vi "WLAN - RxMeasure - DLL - VI.vi"() -> ()   [LabVIEW 2012]
panel:
  out "error out 4":errorcluster
  in  "Path Loss":dbl
  in  "RxPower":dbl
  in  "RF:Frequency (Hz)":dbl
  out "error out 2":errorcluster
  out "error out":errorcluster
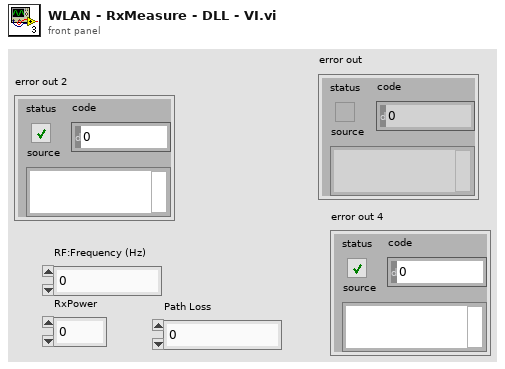
[diagram p1: front panel]
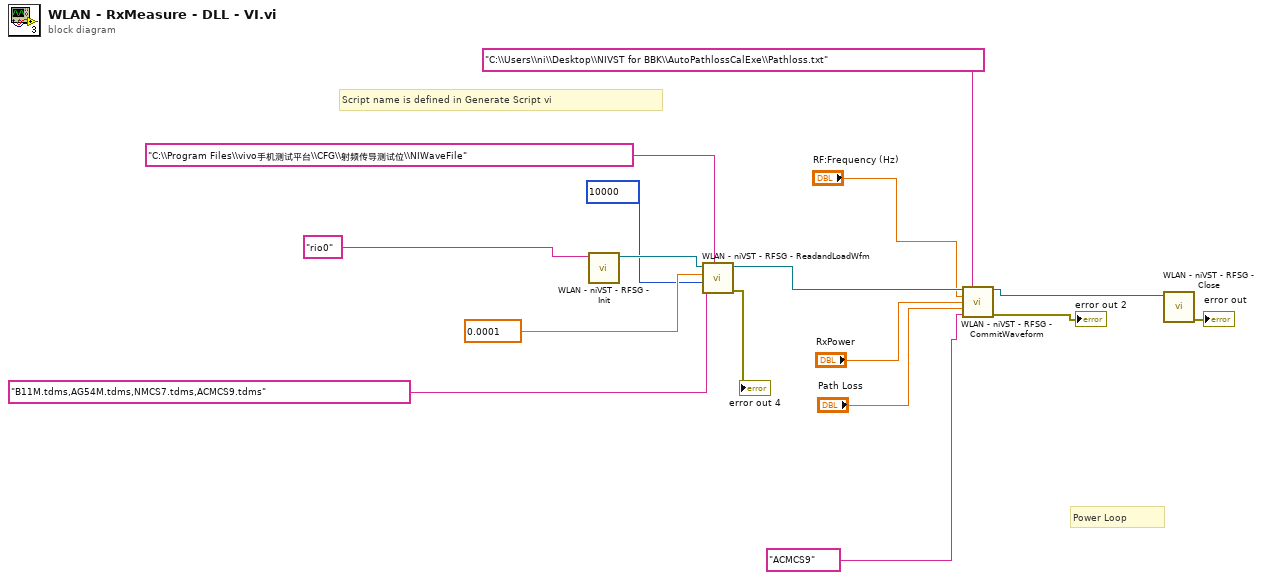
[diagram p0: block diagram]
diagram:
  # "Power Loop"
  # "Script name is defined in Generate Script vi"
  n1 = call "WLAN - niVST - RFSG - Init.vi"("RFSG Handle In"="rio0" ("RFSG Handle")) -> ("RFSG handle Out"=w12:refnum<k15>)  [unwired: 9 in, 1 out]
  n2 = call "WLAN - niVST - RFSG - ReadandLoadWfm.vi"("WfmFolderPath"="C:\\Program Files\\vivo手机测试平台\\CFG\\射频传导测试位\\NIWaveFile", "AllRxWfmName"="B11M.tdms,AG54M.tdms,NMCS7.tdms,ACMCS9.tdms", "numPackets"=10000 ("Number of Packets"), "Idle Time (With Ack)"=0.0001, "RFSG Handle In"=w12) -> ("error out"=→"error out 4":errorcluster, "RFSG Handle Out"=w9:refnum<k15>)  [unwired: 5 in]
  n3 = call "WLAN - niVST - RFSG - CommitWaveform.vi"("RFSG Handle In"=w9, "Internal pathloss file"="C:\\Users\\ni\\Desktop\\NIVST for BBK\\AutoPathlossCalExe\\Pathloss.txt", "RF:Frequency (Hz)"="RF:Frequency (Hz)", "RxPower"="RxPower", "External Path Loss"="Path Loss", "WfmName"="ACMCS9") -> ("RFSG Handle out"=w14:refnum<k15>, "error out"=→"error out 2":errorcluster)  [unwired: 8 in]
  n4 = call "WLAN - niVST - RFSG - Close.vi"("RFSG Handle In"=w14) -> ("error out"=→"error out":errorcluster)  [unwired: 10 in]
